vi "AD原码转物理.vi"(0 "设备句柄入":i32, 1 "原码值":u16[](array[numeric]), 2 "个数":i32, 3 "错误输入":errorcluster caption="错误输入（无错误）") -> (7 "设备句柄":i32=1, 8 "物理值":dbl[](array[numeric]), 10 "错误输出":errorcluster)   [LabVIEW 2016]
uses:
  dll/em9636.dll
panel:
  in  "超时毫秒":i32=1000
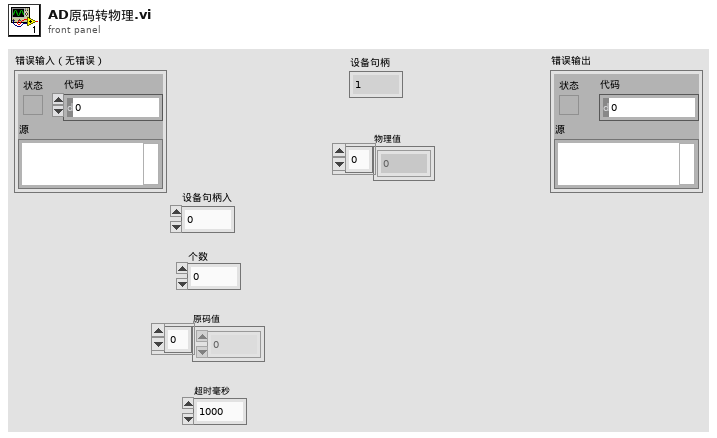
[diagram p1: front panel]
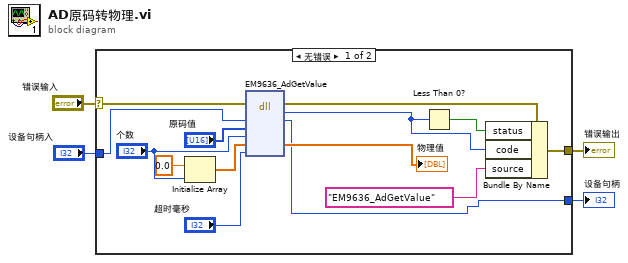
[diagram p0: block diagram]
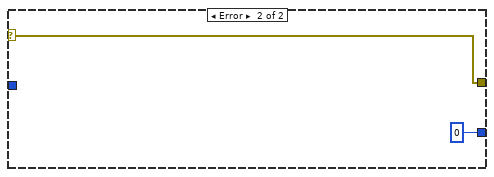
[diagram p2: hidden frame]
diagram:
  n1 = case shown="无错误" "错误输入" {
    selector: "错误输入" -> [w18 w20]
    tunnel: [w14 w20] -> w3
    tunnel: [w5 0 ("错误")] -> w2
    tunnel: "设备句柄入" -> [w12 _]
    frame No Error {
      n2 = Initialize Array(0.0 ("元素"), "个数") -> (w7:dbl[])
      n3 = dll-call lib="PTH2kabs CUsers\nAdministratorDesktopEM9636*EM9636系列_demo_labview(调用DLL方式)dll\nem9636.dll" fn="EM9636_AdGetValue"(error in=w18, "设备句柄"=w12, "原码值"="原码值", "个数"="个数", "物理值"=w7, "超时毫秒"="超时毫秒") -> (error out=w16:errorcluster, "错误"=w13:i32, "设备句柄"=w5:i32, "物理值"=→"物理值":dbl[])  [unwired: 5 in, 1 out]
      n4 = Less Than 0?(x=w13) -> (x < 0?=w15:bool)
      n5 = Bundle By Name(cluster=w16, "status"=w15, "code"=w13, "source"="EM9636_AdGetValue") -> (w14:errorcluster)
    }
    frame Error {
    }
  }
  "错误输出" <- w3
  "设备句柄" <- w2
